vi "HandleExit.vi"(8 "error in (no error)":errorcluster, 9 "VI Refnum":refnum<vi>, 10 "StopArgument":variant, 11 "ModuleAdmin":refnum<class "ModuleAdmin.lvclass">) -> (0 "error out":errorcluster, 1 "Exit via Stop Module Req?":bool, 2 "WaitForStop?":bool)   [LabVIEW 2014, in "WfrmModule.lvlib"]
uses:
  WfrmModule.lvlib
  <userlib>/NIST/ModuleAdminLib/ModuleAdmin/ModuleAdmin.lvclass
  PublicAPI/Arguments/Requests/clStopArgument.ctl
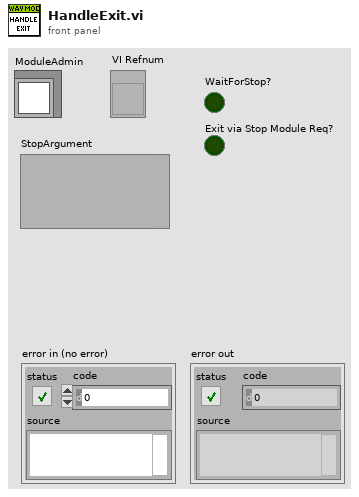
[diagram p1: front panel]
types:
  T1 = typedef "WfrmModule.lvlib/clStopArgument.ctl" = cluster{"Exit via Stop Module Req?":bool, "Wait for Module to stop?":bool, "ModuleAdmin":refnum<class "ModuleAdmin.lvclass">}
  T2 = enum32{"Invalid", "Standard", "Closed", "Hidden", "Minimized", "Maximized"}
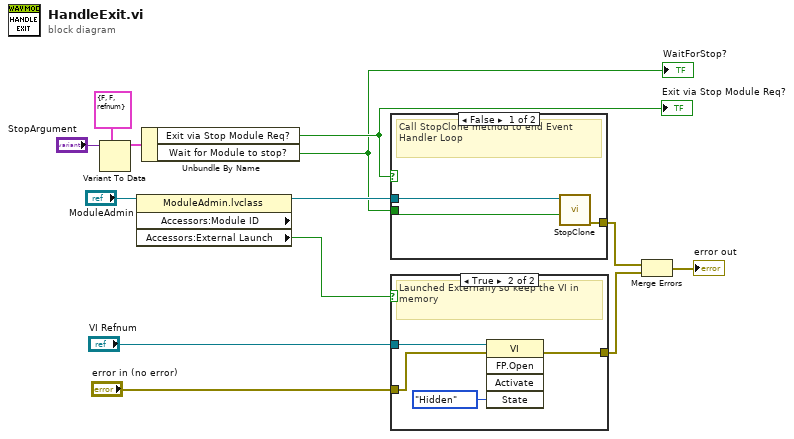
[diagram p0: block diagram]
diagram:
  n1 = Variant To Data(type=T1 {"Exit via Stop Module Req?"=FALSE, "Wait for Module to stop?"=FALSE, "ModuleAdmin"=refnum} ("Stop Argument"), Variant="StopArgument") -> (data=w6:T1)  [unwired: 1 in, 1 out]
  n2 = property class="ModuleAdmin.lvclass" props=["Accessors:Module ID", "Accessors:External Launch"](reference="ModuleAdmin") -> (reference out=w3:refnum<class "ModuleAdmin.lvclass">, "Accessors:External Launch"=w2:bool)  [unwired: 1 in, 2 out]
  n3 = Unbundle By Name(w6) -> ("Exit via Stop Module Req?"=w4:bool, "Wait for Module to stop?"=w1:bool)
  "WaitForStop?" <- w1
  "Exit via Stop Module Req?" <- w4
  n4 = case shown="False" w4 {
    tunnel: [w16 _] -> w10
    tunnel: w1 -> [w15 _]
    tunnel: w3 -> [w14 _]
    frame False {
      # "Call StopClone method to end Event Handler Loop"
      n5 = call "StopClone.vi"("Wait for Module to stop?"=w15, "ModuleAdmin"=w14) -> ("error out"=w16:errorcluster)  [unwired: 9 in]
    }
    frame True {
      # "This came from the Event Handler Loop"
    }
  }
  n6 = case shown="True" w2 {
    tunnel: "VI Refnum" -> [_ w21]
    tunnel: [w17 w19] -> w9
    tunnel: "error in (no error)" -> [w17 w18]
    frame False {
    }
    frame True {
      # "Launched Externally so keep the VI in memory"
      n7 = invoke class="VI" method="FP.Open"(reference=w21, error in=w18, "State"=T2."Hidden") -> (error out=w19:errorcluster)  [unwired: 2 in, 4 out]
    }
  }
  n8 = Merge Errors(w10, w9) -> (→"error out":errorcluster)
